vi "Look up.vi"(8 "column":i32, 9 "row":i32, 10 "Tree":T1, 11 "Array":T1[][](array[typedef])) -> (2 "output cluster":T1)   [LabVIEW 2020]
uses:
  tree--cluster.ctl
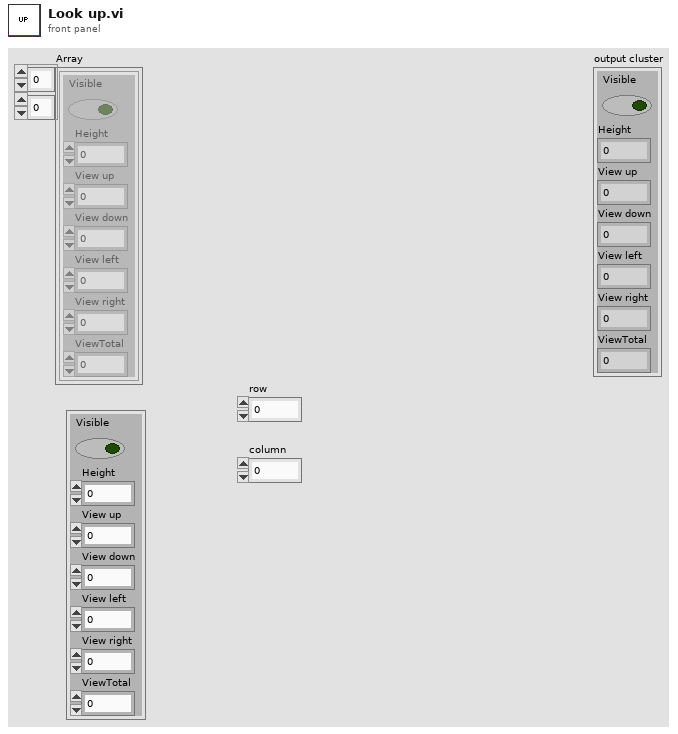
[diagram p1: front panel]
types:
  T1 = typedef "tree--cluster.ctl" = cluster{"Visible":bool, "Height":i32, "View up":i32, "View down":i32, "View left":i32, "View right":i32, "ViewTotal":i32}
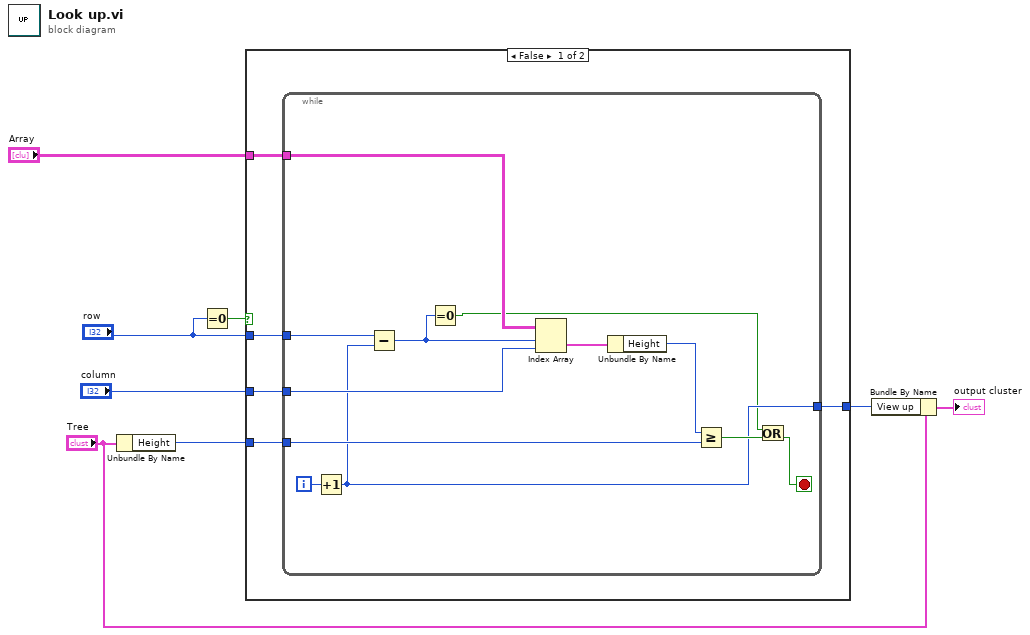
[diagram p0: block diagram]
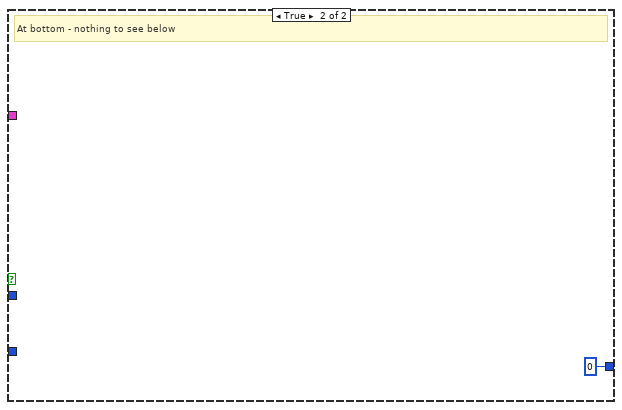
[diagram p2: hidden frame]
diagram:
  n1 = Unbundle By Name("Tree") -> ("Height"=w8:i32)
  n2 = Equal To 0?(x="row") -> (x = 0?=w1:bool)
  n3 = case shown="False" w1 {
    tunnel: w8 -> [w13 _]
    tunnel: "column" -> [w12 _]
    tunnel: "row" -> [w11 _]
    tunnel: [w10 0] -> w5
    tunnel: "Array" -> [w9 _]
    frame False {
      n4 = while {
        tunnel: w13 -> [w19]
        tunnel: w9 -> [w25]
        tunnel: w12 -> [w24]
        tunnel: w11 -> [w23]
        tunnel: [w17] -> w10
        i -> [w22]
        stop <- w15 stop-if-true
        n5 = Increment(x=w22) -> (x+1=w17:i32)
        n6 = Subtract(x=w23, y=w17) -> (x-y=w16:i32)
        n7 = Equal To 0?(x=w16) -> (x = 0?=w14:bool)
        n8 = Index Array(array=w25, index (row)=w16, index (col)=w24) -> (element=w21:T1)
        n9 = Unbundle By Name(w21) -> ("Height"=w20:i32)
        n10 = Greater Or Equal?(x=w20, y=w19) -> (x >= y?=w18:bool)
        n11 = Or(x=w14, y=w18) -> (x .or. y?=w15:bool)
      }
    }
    frame True {
      # "At bottom - nothing to see below"
    }
  }
  n12 = Bundle By Name(cluster="Tree", "View up"=w5) -> (→"output cluster":T1)
